vi "Programming.vi"(8 "error in":errorcluster, 10 "Supply PCB over Programator":bool, 11 "DUT variant":string="327-LEPL-104-M") -> (0 "error out":errorcluster, 1 "Programming passed":bool, 2 "standard error":string, 3 "standard output":string)   [LabVIEW 2023]
panel:
  out "return code":i32
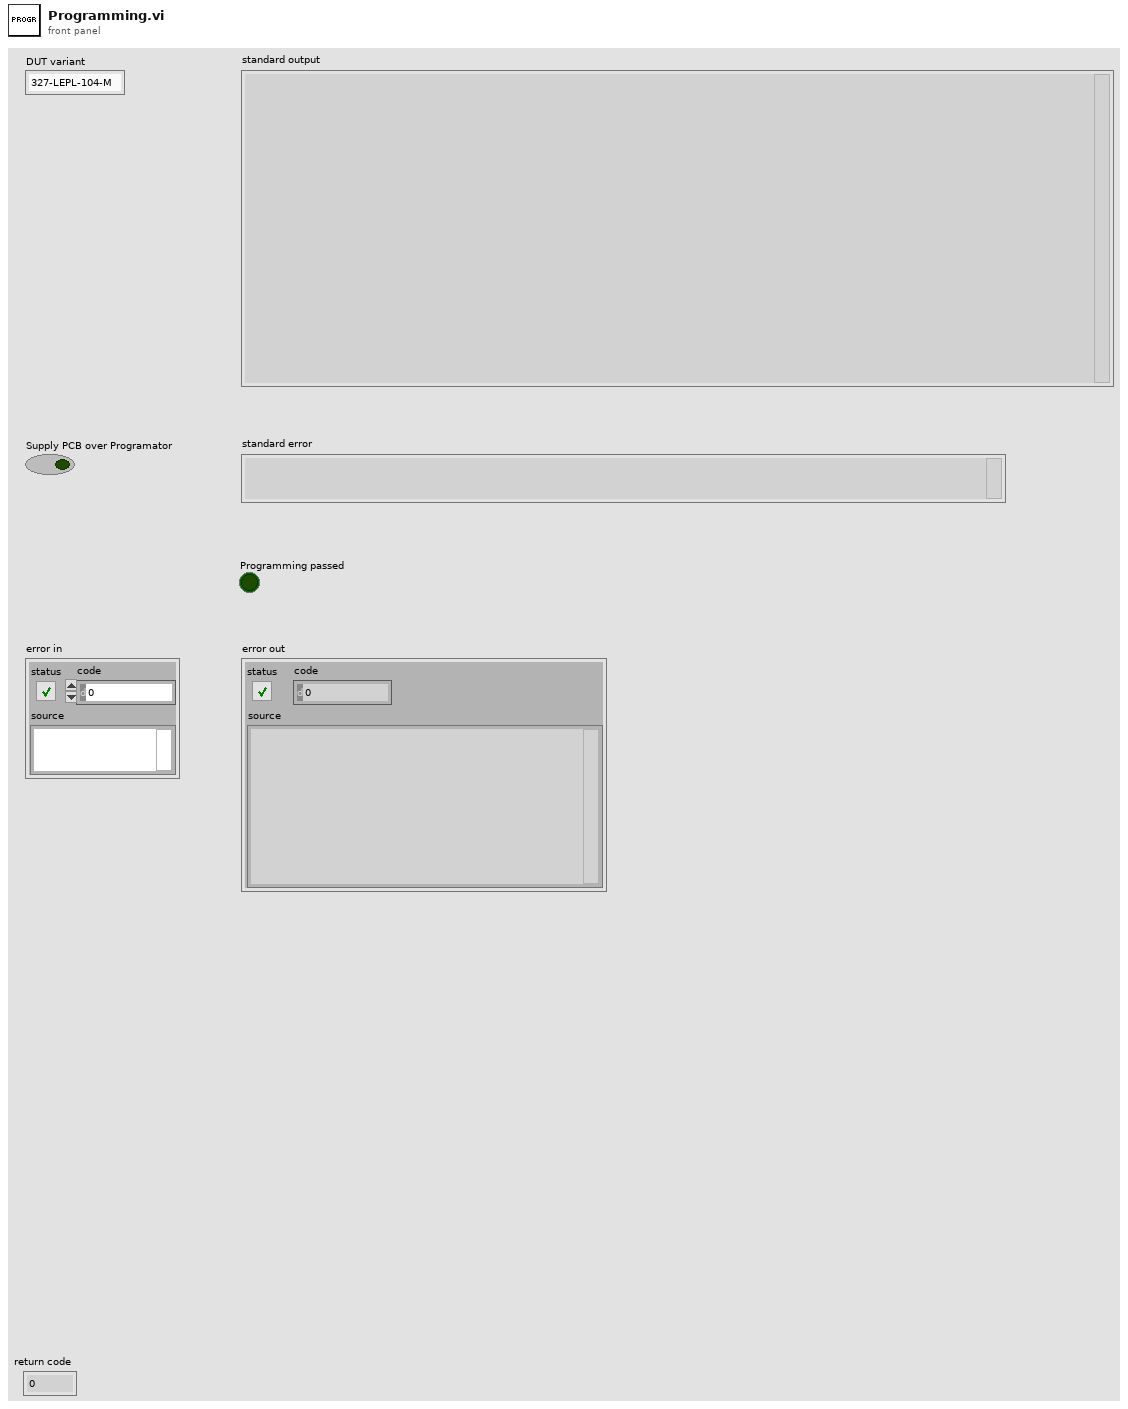
[diagram p1: front panel]
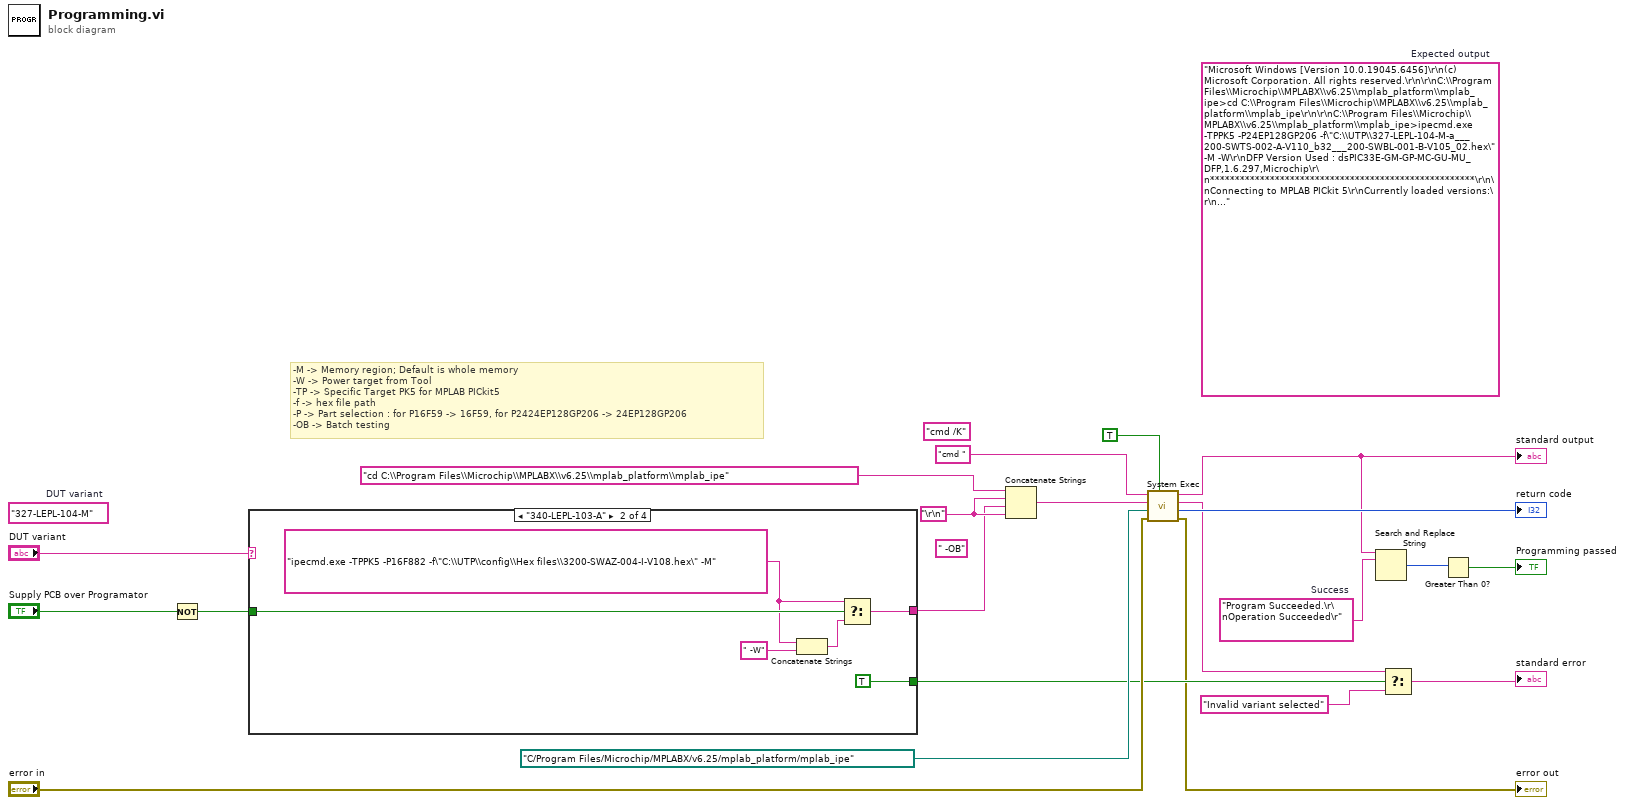
[diagram p0: block diagram]
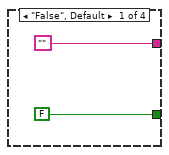
[diagram p2: hidden frame]
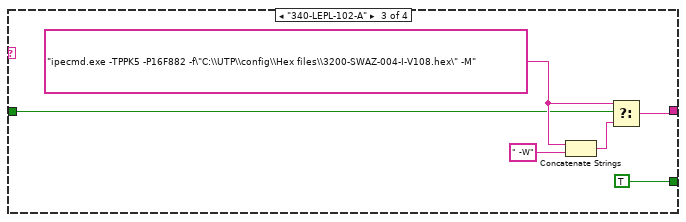
[diagram p3: hidden frame]
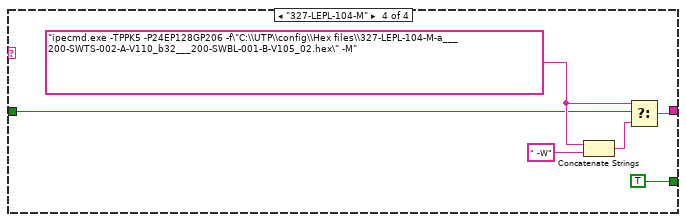
[diagram p4: hidden frame]
diagram:
  (unwired) "cmd /K" ("command line")
  (unwired) " -OB" ("string")
  w6 = "Program Succeeded.\r\nOperation Succeeded\r"  # Success
  (unwired) "Microsoft Windows [Version 10.0.19045.6456]\r\n(c) Microsoft Corporation. All rights reserved.\r\n\r\nC:\\Program Files\\Microchip\\MPLABX\\v6.25\\mplab_platform\\mplab_ipe>cd C:\\Program Files\\Microchip\\MPLABX\\v6.25\\mplab_platform\\mplab_ipe\r\n\r\nC:\\Program Files\\Microchip\\MPLABX\\v6.25\\mplab_platform\\mplab_ipe>ipecmd.exe -TPPK5 -P24EP128GP206 -f\"C:\\UTP\\327-LEPL-104-M-a___200-SWTS-002-A-V110_b32___200-SWBL-001-B-V105_02.hex\" -M -W\r\nDFP Version Used : dsPIC33E-GM-GP-MC-GU-MU_DFP,1.6.297,Microchip\r\n*****************************************************\r\n\nConnecting to MPLAB PICkit 5\r\nCurrently loaded versions:\r\nApplication version...........02.04.54\r\nBoot version..................00.00.68\r\nPCB version...................3\r\nScript version................00.08.91\r\nScript build number...........0674c1b56b\r\nTool pack version ............2.9.699\r\nBLE version ..................1.44\r\nPICkit 5 is supplying power to the target (3.25 volts).\r\nTarget device PIC24EP128GP206 found.\r\nDevice Revision Id  = 0x4008\r\nDevice Id = 0x1e5b0000\r\n*****************************************************\r\nCalculating memory ranges for operation...\r\nErasing...\r\nThe following memory area(s) will be programmed:\r\nprogram memory: start address = 0x0, end address = 0x7ff\nprogram memory: start address = 0x1000, end address = 0x97ff\nprogram memory: start address = 0x13800, end address = 0x13fff\nprogram memory: start address = 0x14800, end address = 0x157eb\nconfiguration memory\nUser Id Memory\r\nProgramming/Verify complete\r\n Program Report\r\n2026-01-16, 11:57:39\r\nDevice Type:PIC24EP128GP206\r\nProgram Succeeded.\r\nOperation Succeeded\r\n\r\nC:\\Program Files\\Microchip\\MPLABX\\v6.25\\mplab_platform\\mplab_ipe>"  # Expected output
  (unwired) "327-LEPL-104-M"  # DUT variant
  w2 = "\r\n"
  # "-M -> Memory region; Default is whole memory\n-W -> Power target from Tool\n-TP -> Specific Target PK5 for MPLAB PICkit5\n-f -> hex file path\n-P -> Part selection : for P16F59 -> 16F59, for P2424EP128GP206 -> 24EP128GP206\n-OB -> Batch testing"
  n1 = Not(x="Supply PCB over Programator") -> (.not. x?=w13:bool)
  n2 = case shown="\"340-LEPL-103-A\"" "DUT variant" {
    tunnel: ["" w25 w32 w38] -> w1
    tunnel: w13 -> [_ w28 w31 w37]
    tunnel: [FALSE ("s") TRUE ("s") TRUE ("s") TRUE ("s")] -> w11
    frame "False", Default {
    }
    frame "340-LEPL-103-A" {
      w27 = "ipecmd.exe -TPPK5 -P16F882 -f\"C:\\UTP\\config\\Hex files\\3200-SWAZ-004-I-V108.hex\" -M" ("command line")
      n3 = Concatenate Strings(w27, " -W" ("string")) -> (w26:string)
      n4 = Select(t=w27, s=w28, f=w26) -> (s? t:f=w25:string)
    }
    frame "340-LEPL-102-A" {
      w33 = "ipecmd.exe -TPPK5 -P16F882 -f\"C:\\UTP\\config\\Hex files\\3200-SWAZ-004-I-V108.hex\" -M" ("command line")
      n5 = Concatenate Strings(w33, " -W" ("string")) -> (w34:string)
      n6 = Select(t=w33, s=w31, f=w34) -> (s? t:f=w32:string)
    }
    frame "327-LEPL-104-M" {
      w39 = "ipecmd.exe -TPPK5 -P24EP128GP206 -f\"C:\\UTP\\config\\Hex files\\327-LEPL-104-M-a___200-SWTS-002-A-V110_b32___200-SWBL-001-B-V105_02.hex\" -M" ("command line")
      n7 = Concatenate Strings(w39, " -W" ("string")) -> (w40:string)
      n8 = Select(t=w39, s=w37, f=w40) -> (s? t:f=w38:string)
    }
  }
  n9 = Concatenate Strings("cd C:\\Program Files\\Microchip\\MPLABX\\v6.25\\mplab_platform\\mplab_ipe" ("command line"), w2, w1, w2) -> (w17:string)
  n10 = call <vilib>:"System Exec.vi"("wait until completion? (T)"=TRUE, "error in (no error)"="error in", "working directory"=path "C:/Program Files/Microchip/MPLABX/v6.25/mplab_platform/mplab_ipe", "standard input"=w17, "command line"="cmd ") -> ("error out"=→"error out":errorcluster, "return code"=→"return code":i32, "standard error"=w9:string, "standard output"=w7:string)  [unwired: 3 in]
  "standard output" <- w7
  n11 = Search and Replace String(input string=w7, search string=w6) -> (number of replacements=w5:i32)  [unwired: 6 in, 3 out]
  n12 = Select(t=w9, s=w11, f="Invalid variant selected") -> (s? t:f=→"standard error":string)
  n13 = Greater Than 0?(x=w5) -> (x > 0?=→"Programming passed":bool)
